vi "sslSimulationProtocolDecodeRobotFeedback.vi"(8 "error in (no error)":errorcluster, 11 "robotFeedbackArray":u8[](array[numeric])) -> (0 "error out":errorcluster, 3 "RobotFeedback.lvclass":refnum<class "RobotFeedback.lvclass">)   [LabVIEW 2021, in "Communication.lvclass"]
uses:
  Communication.lvclass
  RobotFeedback/RobotFeedback.lvclass
  feedbackData.ctl
  RobotFeedback/Write id.vi
  RobotFeedback/Write dribblerContactToBall.vi
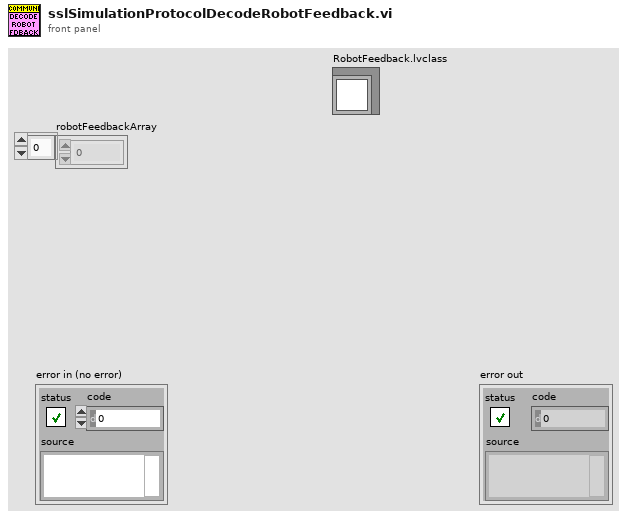
[diagram p1: front panel]
types:
  T1 = typedef "feedbackData.ctl" = cluster{"id":u32, "status":u32, "battery":sgl, "encoder1":sgl, "encoder2":sgl, "encoder3":sgl, "encoder4":sgl}
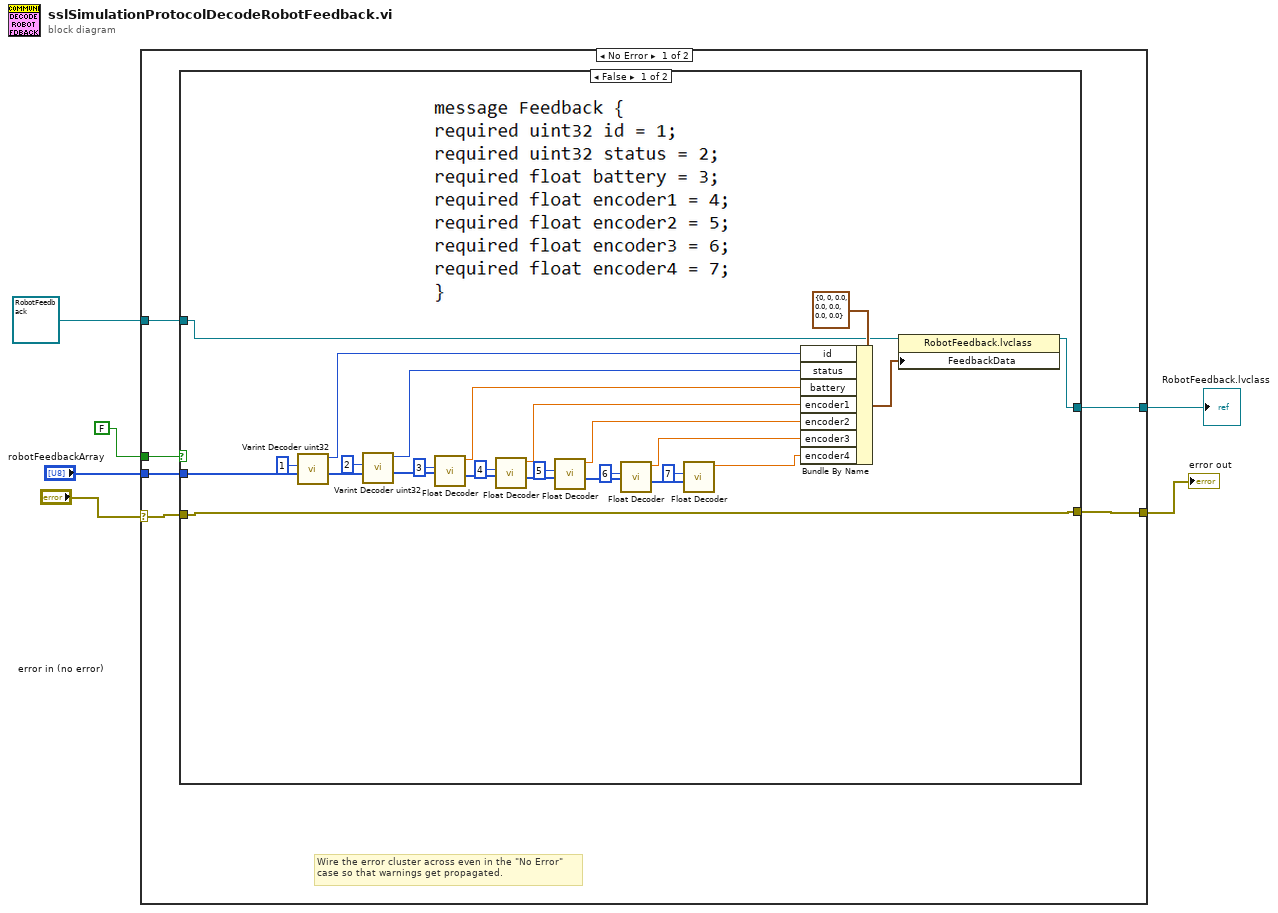
[diagram p0: block diagram]
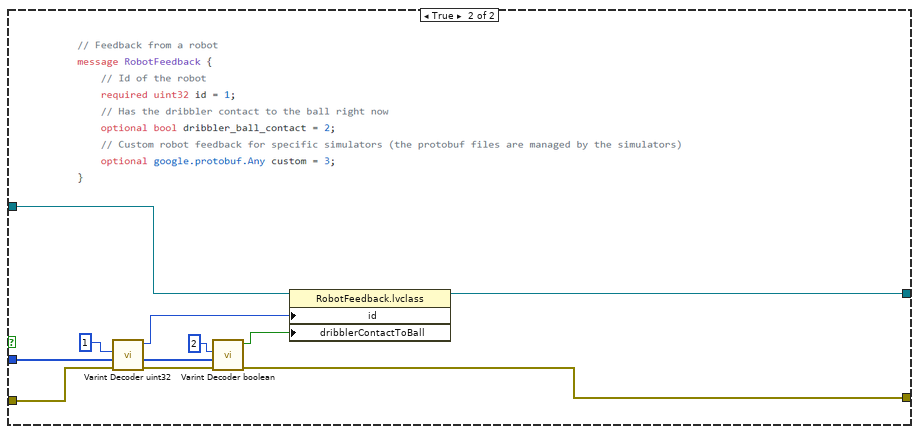
[diagram p2: hidden frame]
diagram:
  n1 = case shown="No Error" "error in (no error)" {
    selector: "error in (no error)" -> [w11 w50]
    tunnel: [w10 w50] -> w5
    tunnel: "robotFeedbackArray" -> [w12 _]
    tunnel: refnum<class "RobotFeedback.lvclass"> refnum ("RobotFeedback.lvclass") -> [w9 _]
    tunnel: [w8 _] -> w2
    tunnel: FALSE -> [w7 _]
    frame No Error {
      # "Wire the error cluster across even in the \"No Error\"\ncase so that warnings get propagated."
      n2 = case shown="False" w7 {
        tunnel: w12 -> [w38 w49]
        tunnel: w11 -> [w15 w44]
        tunnel: [w15 w43] -> w10
        tunnel: w9 -> [w14 w42]
        tunnel: [w16 w39] -> w8
        frame False {
          n3 = call "Varint Decoder uint32.vi"("Array"=w38, "Key"=1) -> ("array w/ subset deleted"=w36:u8[], "Varint"=w13:u32)  [unwired: 6 in, 2 out]
          n4 = call "Varint Decoder uint32.vi"("Array"=w36, "Key"=2) -> ("array w/ subset deleted"=w34:u8[], "Varint"=w22:u32)  [unwired: 6 in, 2 out]
          n5 = call "Float Decoder.vi"("Array"=w34, "Key"=3) -> ("array w/ subset deleted"=w32:u8[], "Float"=w21:sgl)  [unwired: 6 in, 2 out]
          n6 = call "Float Decoder.vi"("Array"=w32, "Key"=4) -> ("array w/ subset deleted"=w30:u8[], "Float"=w20:sgl)  [unwired: 6 in, 2 out]
          n7 = call "Float Decoder.vi"("Array"=w30, "Key"=5) -> ("array w/ subset deleted"=w29:u8[], "Float"=w19:sgl)  [unwired: 6 in, 2 out]
          n8 = call "Float Decoder.vi"("Array"=w29, "Key"=6) -> ("array w/ subset deleted"=w28:u8[], "Float"=w18:sgl)  [unwired: 6 in, 2 out]
          n9 = call "Float Decoder.vi"("Array"=w28, "Key"=7) -> ("Float"=w17:sgl)  [unwired: 6 in, 3 out]
          n10 = Bundle By Name(cluster=T1 {"id"=0, "status"=0, "battery"=0.0, "encoder1"=0.0, "encoder2"=0.0, "encoder3"=0.0, "encoder4"=0.0} ("FeedbackData"), "id"=w13, "status"=w22, "battery"=w21, "encoder1"=w20, "encoder2"=w19, "encoder3"=w18, "encoder4"=w17) -> (w23:T1)
          n11 = property class="RobotFeedback.lvclass"(reference=w14, "FeedbackData"=w23) -> (reference out=w16:refnum<class "RobotFeedback.lvclass">)  [unwired: 1 in, 1 out]
        }
        frame True {
          n12 = call "Varint Decoder uint32.vi"("error in (no error)"=w44, "Array"=w49, "Key"=1) -> ("error out"=w45:errorcluster, "array w/ subset deleted"=w47:u8[], "Varint"=w41:u32)  [unwired: 5 in, 1 out]
          n13 = call "Varint Decoder boolean.vi"("error in (no error)"=w45, "Array"=w47, "Key"=2) -> ("error out"=w43:errorcluster, "bool"=w40:bool)  [unwired: 5 in, 2 out]
          n14 = property class="RobotFeedback.lvclass"(reference=w42, "id"=w41, "dribblerContactToBall"=w40) -> (reference out=w39:refnum<class "RobotFeedback.lvclass">)  [unwired: 1 in, 1 out]
        }
      }
    }
    frame Error {
    }
  }
  "error out" <- w5
  "RobotFeedback.lvclass" <- w2
